vi "VoltageTest_L_VDC9V.vi"(0 "datain":string[](array[string])=["备注", "负载通道", "负载地址", "延时时间", "output max", "output min", "量测类型", "待测物板号"], 5 "HW CH Number":i32, 7 "Setup":string) -> (4 "REPORT INDECATE":string[][](array[string])=[["微安测试", "", "", "", ""], ["微安量测", "4", "0.000", "0.1", "NG"], ["微安量测", "4", "0.000", "0.1", "NG"], ["微安量测", "4", "0.000", "0.1", "NG"], ["微安量测", "4", "0.000", "0.1", "NG"]], 6 "ROW HEAD":string[](array[string]), 8 "PF":string[](array[string]), 10 "testData":string[](array[string]), 15 "Array":string[](array[string]))   [LabVIEW 2018]
uses:
  Subvi/Global.vi
panel:
  out "元素":string
  out "测试板数":i32
  out "数组":bool[](array[boolean])
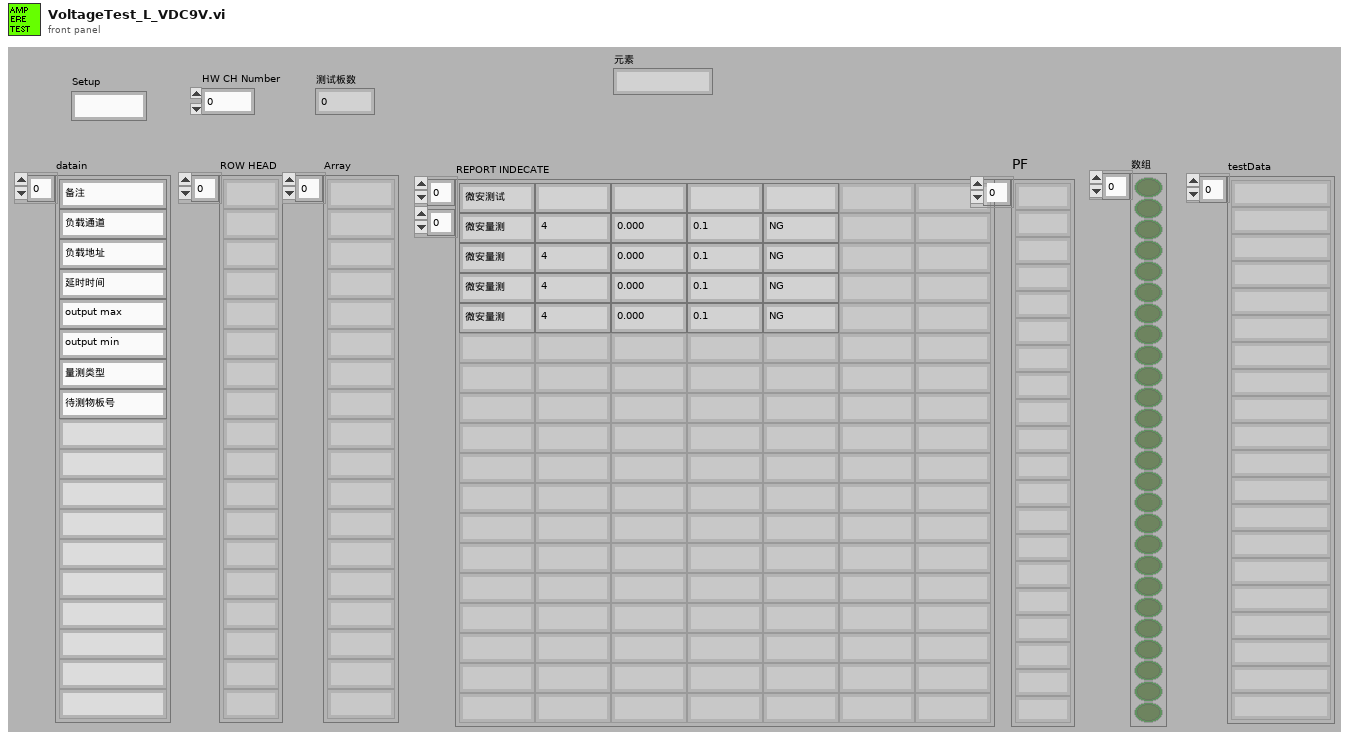
[diagram p1: front panel]
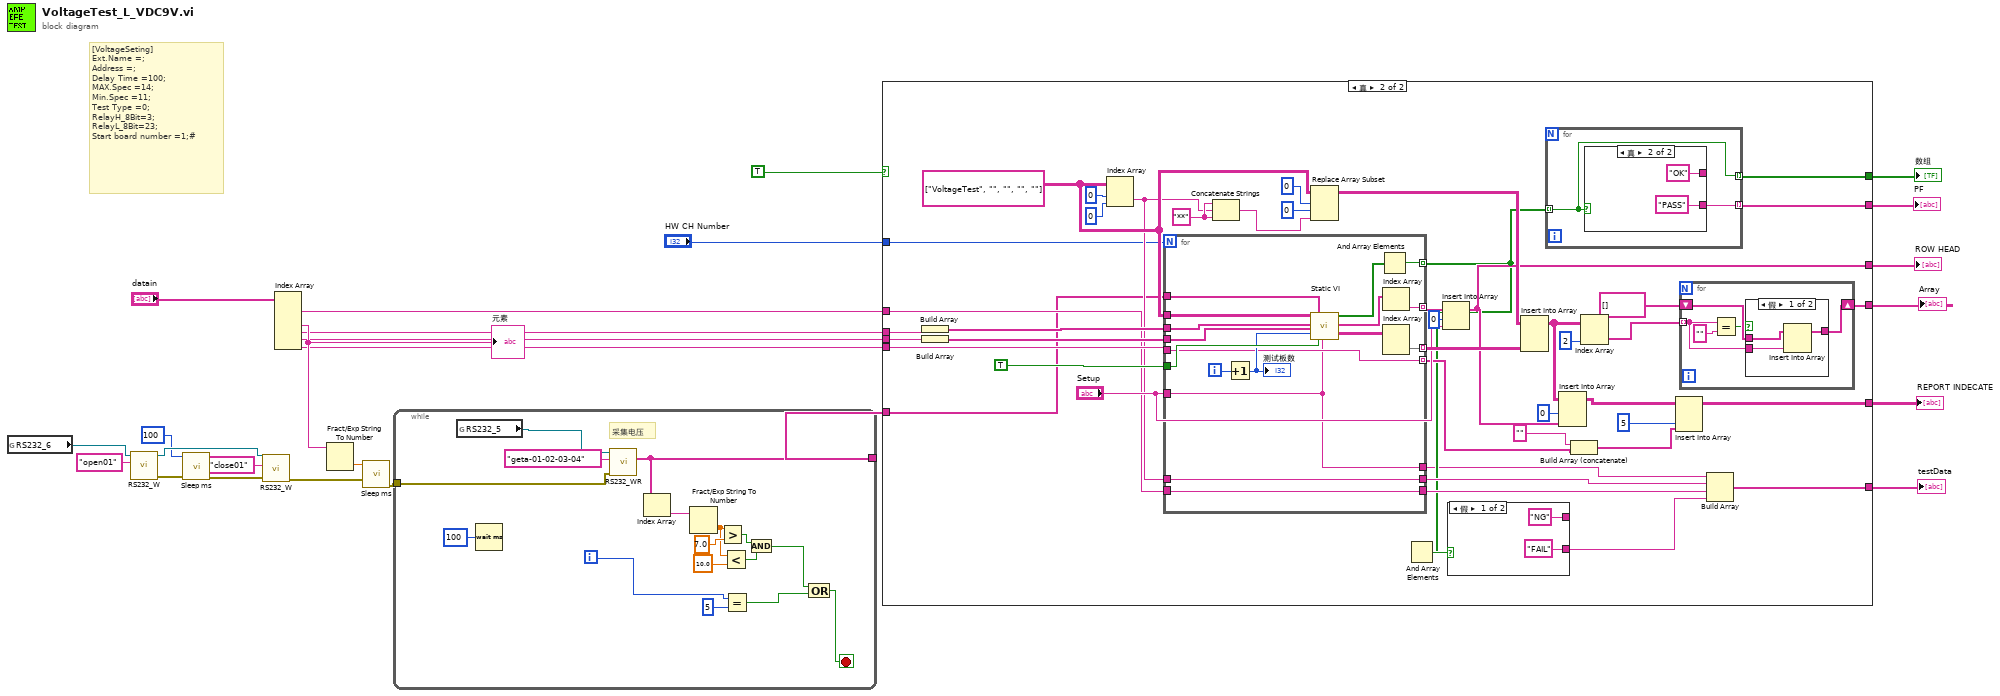
[diagram p0: block diagram]
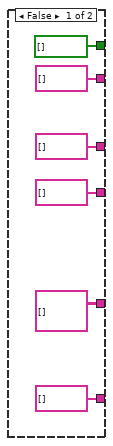
[diagram p2: hidden frame]
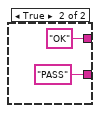
[diagram p3: hidden frame]
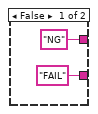
[diagram p4: hidden frame]
diagram:
  # "[VoltageSeting]\nExt.Name =;\nAddress =;\nDelay Time =100;\nMAX.Spec =14;\nMin.Spec =11;\nTest Type =0;\nRelayH_8Bit=3;\nRelayL_8Bit=23;\nStart board number =1;#"
  n1 = global read "Global.vi" "RS232_6"() -> (w10:refnum<visa-resource-name>)
  n2 = call "RS232_W.vi"("CMD"="open01", "VISA资源名称"=w10) -> ("error out"=w7:errorcluster, "VISA资源名称输出"=w9:refnum<visa-resource-name>)  [unwired: 7 in, 1 out]
  n3 = call "Sleep ms.vi"("error in (no error)"=w7, "等待时间（毫秒）"=u32 100) -> ("error out"=w8:errorcluster)  [unwired: 9 in]
  n4 = call "RS232_W.vi"("error in (no error)"=w8, "CMD"="close01", "VISA资源名称"=w9) -> ("error out"=w2:errorcluster)  [unwired: 6 in, 2 out]
  n5 = Index Array(array="datain") -> (element #1=w16:string, element #3=w22:string, element #4=w21:string, element #5=w20:string, element #6=w18:string)  [unwired: 6 in, 1 out]
  "元素" <- w22
  n6 = Fract/Exp String To Number(string=w22) -> (number=w3:dbl)  [unwired: 3 in, 1 out]
  n7 = call "Sleep ms.vi"("error in (no error)"=w2, "等待时间（毫秒）"=w3) -> ("error out"=w1:errorcluster)  [unwired: 9 in]
  n8 = while {
    tunnel: [w29] -> w12
    tunnel: w1 -> [w27]
    i -> [w31]
    stop <- w30 stop-if-true
    # "采集电压"
    n9 = global read "Global.vi" "RS232_5"() -> (w40:refnum<visa-resource-name>)
    n10 = Wait (ms)(milliseconds to wait=u32 100 ("等待时间（毫秒）")) -> ()  [unwired: 1 out]
    n11 = call "RS232_WR.vi"("error in (no error)"=w27, "CMD"="geta-01-02-03-04", "VISA资源名称"=w40) -> ("Out data"=w29:string[])  [unwired: 6 in, 2 out]
    n12 = Index Array(array=w29) -> (element=w28:string)  [unwired: 1 in]
    n13 = Fract/Exp String To Number(string=w28) -> (number=w33:dbl)  [unwired: 3 in, 1 out]
    n14 = Greater?(x=w33, y=7.0) -> (0:w35:bool)
    n15 = Less?(x=w33, y=10.0) -> (x < y?=w36:bool)
    n16 = Equal?(x=w31, y=5) -> (x = y?=w39:bool)
    n17 = And(x=w35, y=w36) -> (x .and. y?=w34:bool)
    n18 = Compound Arithmetic op=OR ("复合运算")(w34, w39) -> (w30:bool)
  }
  n19 = case shown="真" TRUE {
    tunnel: [string[] [] ("Array") w88] -> w25
    tunnel: [string[] [] w87] -> w24
    tunnel: w21 -> [_ w80]
    tunnel: w20 -> [_ w79]
    tunnel: [string[] [] w68] -> w19
    tunnel: w18 -> [_ w66]
    tunnel: [string[][] [] w63] -> w17
    tunnel: w16 -> [_ w58]
    tunnel: [string[] [] w52] -> w15
    tunnel: [bool[] [] w50] -> w14
    tunnel: "HW CH Number" -> [_ w49]
    tunnel: w12 -> [_ w48]
    frame False {
    }
    frame True {
      w78 = string[][] [["VoltageTest", "", "", "", ""]]
      w84 = "**" ("字符串")
      n20 = Build Array(w80) -> (w77:string[])
      n21 = Build Array(w79) -> (w76:string[])
      n22 = Index Array(array=w78, index (row)=0 ("索引 (行)"), index (col)=0 ("禁用的索引 (列)")) -> (element=w59:string)
      n23 = for {
        N: w49 -> [_]
        tunnel: w48 -> [w112]
        tunnel: w77 -> [w110]
        tunnel: w76 -> [w109]
        tunnel: "Setup" -> [w96]
        tunnel: TRUE -> [w107]
        tunnel: [w105] -> w54 mode=indexing
        tunnel: [w102] -> w72 mode=indexing
        tunnel: w78 -> [w111]
        tunnel: [w100] -> w73 mode=indexing
        tunnel: w66 -> [w99]
        tunnel: [w99] -> w62 mode=indexing
        tunnel: w59 -> [w98]
        tunnel: [w98] -> w57
        tunnel: w58 -> [w97]
        tunnel: [w97] -> w56
        tunnel: [w96] -> w51
        i -> [w104]
        n24 = Increment(x=w104) -> (x+1=w106:i32)
        "测试板数" <- w106
        n25 = call "Static VI.vi"("添加的数组"=w111, "Max"=w110, "Min"=w109, "板数"=w106, "INPUTSTRING"=w112, "是否为字符串对比"=w107, "SQ"=w96) -> ("P/F"=w108:bool[], "SQ out"=w103:string[], "arrauy out"=w101:string[][])  [unwired: 9 in, 1 out]
        n26 = And Array Elements(Boolean array=w108) -> (logical AND=w105:bool)
        n27 = Index Array(array=w103) -> (element=w102:string)  [unwired: 1 in]
        n28 = Index Array(array=w101) -> (element=w100:string[])  [unwired: 2 in]
      }
      n29 = Concatenate Strings(w84, w59, w84) -> (w81:string)
      n30 = Replace Array Subset(array=w78, new element=w81, index (row)=0 ("索引 (行)"), index (col)=0 ("禁用的索引 (列)")) -> (w74:string[][])
      n31 = And Array Elements(Boolean array=w54) -> (logical AND=w55:bool)
      n32 = Insert Into Array(array=w72, index=0 ("索引"), new element="Setup") -> (w68:string[])
      n33 = case shown="假" w55 {
        tunnel: ["NG" "OK"] -> _
        tunnel: ["FAIL" "PASS"] -> w53
        frame False {
        }
        frame True {
        }
      }
      n34 = Insert Into Array ("数组插入")(array=w74, new element=w73) -> (w69:string[][])  [unwired: 2 in]
      n35 = for {
        tunnel: w54 -> [w113] mode=indexing
        tunnel: [w114] -> w87 mode=indexing
        tunnel: [w113] -> w50 mode=indexing
        n36 = case shown="真" w113 {
          tunnel: ["NG" "OK"] -> _
          tunnel: ["FAIL" "PASS"] -> w114
          frame False {
          }
          frame True {
          }
        }
      }
      n37 = Insert Into Array(array=w69, index (col)=0 ("禁用的索引 (列)"), new element=w68) -> (w64:string[][])  [unwired: 1 in]
      n38 = Build Array (concatenate)("" ("字符串"), w62) -> (w60:string[])
      n39 = Index Array(array=w69, index (col)=2 ("禁用的索引 (列)")) -> (element=w89:string[])  [unwired: 1 in]
      n40 = Insert Into Array(array=w64, index (col)=5 ("禁用的索引 (列)"), new element=w60) -> (w63:string[][])  [unwired: 1 in]
      n41 = for {
        tunnel: w89 -> [w119] mode=indexing
        shift-right: [w120] -> w88
        shift-left: string[] [] ("Array") -> [w123]
        n42 = Equal?(x=w119, y="") -> (x = y?=w121:bool)
        n43 = case shown="假" w121 {
          tunnel: w123 -> [w126 w127]
          tunnel: [w125 w127] -> w120
          tunnel: w119 -> [w124 _]
          frame False {
            n44 = Insert Into Array(array=w126, new element=w124) -> (w125:string[])  [unwired: 1 in]
          }
          frame True {
          }
        }
      }
      n45 = Build Array(w51, w57, w56, w53) -> (w52:string[])
    }
  }
  "REPORT INDECATE" <- w17
  "ROW HEAD" <- w19
  "PF" <- w24
  "Array" <- w25
  "数组" <- w14
  "testData" <- w15
